vi "connect PG server.vi"(8 "error in (no error)":errorcluster, 11 "SP in":refnum<class "PG messages.lvclass">) -> (0 "error out":errorcluster, 2 "conn_out":u64, 3 "SP out":refnum<class "PG messages.lvclass">)   [LabVIEW 2019, in "PG messages.lvclass"]
uses:
  PG messages.lvclass
  D:/my_projects/projects/Algorithms/Labview/19/Database/Save messages PGserver/Save messages PGserver.lvclass
  Save messages PGserver/Save messages PGserver.lvclass/Save messages PGserver.ctl
  PostgreSQL2LabVIEW/libpqlv/src/PQfinish.vi
  PostgreSQL2LabVIEW/libpqlv/src/PQconnectdb.vi
  PostgreSQL2LabVIEW/libpqlv/src/PQerrorMessage.vi
  PostgreSQL2LabVIEW/libpqlv/src/PQstatus.vi
  <vilib>/dlg_ctls.llb/Space Constant.vi
  PostgreSQL2LabVIEW/libpqUtility/src/PQexecute.vi
  PostgreSQL2LabVIEW/libpqUtility/src/PQlistSequenses.vi
  PostgreSQL2LabVIEW/libpqlv/src/PQresultErrorMessage.vi
  PostgreSQL2LabVIEW/libpqUtility/src/PQclear.vi
  PostgreSQL2LabVIEW/libpqlv/src/PQsendQuery.vi
  PostgreSQL2LabVIEW/libpqlv/src/PQgetResult.vi
  PostgreSQL2LabVIEW/libpqlv/src/PQresultStatus.vi
  PostgreSQL2LabVIEW/libpqUtility/src/PQgetColumn.vi
  PostgreSQL2LabVIEW/libpqlv/src/PQclear.vi
  PostgreSQL2LabVIEW/libpqUtility/src/PQfetchTables.vi
  PostgreSQL2LabVIEW/libpqlv/src/PQgetvalue.vi
  PostgreSQL2LabVIEW/libpqlv/src/PQntuples.vi
  PostgreSQL2LabVIEW/libpqUtility64/libpqutility64.lvlib
  PostgreSQL.lvlib
  Save messages PGserver/Save messages PGserver.lvclass
  PostgreSQL2LabVIEW/libpqUtility/libpqutility.lvlib
panel:
  out "PQStatus":T1(ring)
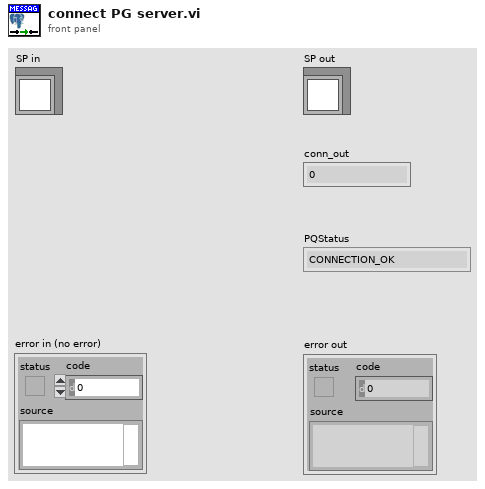
[diagram p1: front panel]
types:
  T1 = enum32{"CONNECTION_OK", "CONNECTION_BAD", "CONNECTION_STARTED", "CONNECTION_MADE", "CONNECTION_AWAITING_RESPONSE", "CONNECTION_AUTH_OK", "CONNECTION_SETENV", "CONNECTION_SSL_STARTUP", "CONNECTION_NEEDED"}
  T2 = typedef "PostgreSQL.lvlib/Coninfo.ctl" = cluster{"host":string, "port":string, "client_encoding":string, "dbname":string, "user":string, "password":string}
  T3 = typedef "Save messages PGserver.lvclass/table parameters.ctl" = cluster{"table postfix":string, "sequence name":string, "columns name":string[], "columns type":string}
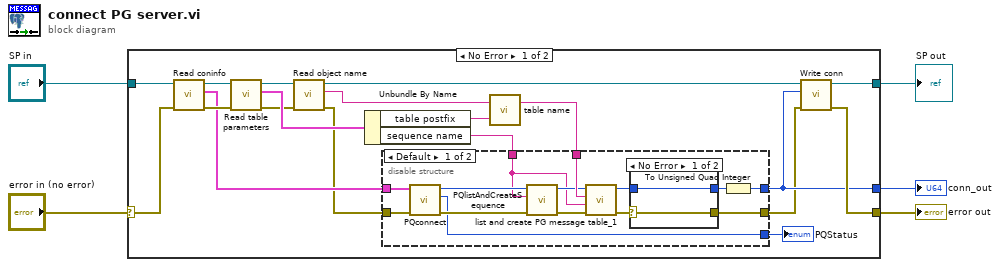
[diagram p0: block diagram]
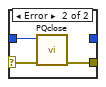
[diagram p2: hidden frame]
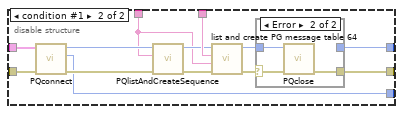
[diagram p3: hidden frame]
diagram:
  n1 = case shown="No Error" "error in (no error)" {
    selector: "error in (no error)" -> [w21 w62]
    tunnel: [w19 w62] -> w4
    tunnel: [w20 w63] -> w2
    tunnel: "SP in" -> [w24 w63]
    tunnel: [w8 _] -> w1
    frame No Error {
      n2 = call "Read coninfo.vi"("error in (no error)"=w21, "SP in"=w24) -> ("error out"=w23:errorcluster, "conninfo"=w10:T2, "SP out"=w22:refnum<class "PG messages.lvclass">)  [unwired: 7 in]
      n3 = call "Read table parameters.vi"("error in (no error)"=w23, "SP in"=w22) -> ("error out"=w12:errorcluster, "table parameters"=w17:T3, "SP out"=w14:refnum<class "PG messages.lvclass">)  [unwired: 7 in]
      n4 = call "Read object name.vi"("error in (no error)"=w12, "SP in"=w14) -> ("error out"=w9:errorcluster, "object name"=w11:string, "SP out"=w13:refnum<class "PG messages.lvclass">)  [unwired: 7 in]
      n5 = Unbundle By Name(w17) -> ("table postfix"=w16:string, "sequence name"=w15:string)
      n6 = call "table name.vi"("postfix"=w16, "object name"=w11) -> ("table name"=w18:string)  [unwired: 1 in]
      n7 = disable-structure shown="Default" {
        disable-tunnel: w18 -> [w38 w56]
        disable-tunnel: w15 -> [w25 w44]
        disable-tunnel: w10 -> [w35 w53]
        disable-tunnel: w9 -> [w34 w52]
        disable-tunnel: [w26 w47] -> w8
        disable-tunnel: [w28 w46] -> w7
        disable-tunnel: [w27 w45] -> w6
        frame condition #0 (active) {
          n8 = call "PQconnect.vi"("error in (no error)"=w34, "conninfo"=w35) -> ("error out"=w32:errorcluster, "PQStatus"=w27:T1, "conn"=w33:u32)  [unwired: 7 in]
          n9 = call "PQlistAndCreateSequence.vi"("error in"=w32, "sequence name"=w25, "conn"=w33) -> ("error out"=w36:errorcluster, "conn_out"=w37:u32)  [unwired: 7 in]
          n10 = call "list and create PG message table_1.vi"("error in"=w36, "serial_n name"=w25, "table name"=w38, "conn"=w37) -> ("error out"=w30:errorcluster, "conn_out"=w31:u32)  [unwired: 6 in]
          n11 = case shown="No Error" w30 {
            selector: w30 -> [w39 w42]
            tunnel: w31 -> [w40 w43]
            tunnel: [w40 _] -> w29
            tunnel: [w39 w41] -> w28
            frame No Error {
            }
            frame Error {
              n12 = call "PQclose.vi"("error in (no error)"=w42, "conn"=w43) -> ("error out"=w41:errorcluster)  [unwired: 9 in]
            }
          }
          n13 = To Unsigned Quad Integer(1:w29) -> (0:w26:u64)
        }
        frame condition #1 {
          n14 = call "PQconnect.vi"("error in (no error)"=w52, "conninfo"=w53) -> ("error out"=w50:errorcluster, "PQStatus"=w45:T1, "conn"=w51:u64)  [unwired: 7 in]
          n15 = call "PQlistAndCreateSequence.vi"("error in"=w50, "sequence name"=w44, "conn"=w51) -> ("error out"=w54:errorcluster, "conn_out"=w55:u64)  [unwired: 7 in]
          n16 = call "list and create PG message table 64.vi"("error in"=w54, "serial_n name"=w44, "table name"=w56, "conn"=w55) -> ("error out"=w48:errorcluster, "conn_out"=w49:u64)  [unwired: 6 in]
          n17 = case shown="Error" w48 {
            selector: w48 -> [w57 w60]
            tunnel: w49 -> [w58 w61]
            tunnel: [w58 _] -> w47
            tunnel: [w57 w59] -> w46
            frame No Error {
            }
            frame Error {
              n18 = call "PQclose.vi"("error in (no error)"=w60, "conn"=w61) -> ("error out"=w59:errorcluster)  [unwired: 9 in]
            }
          }
        }
      }
      "PQStatus" <- w6
      n19 = call "Write conn.vi"("error in (no error)"=w7, "conn"=w8, "SP in"=w13) -> ("error out"=w19:errorcluster, "SP out"=w20:refnum<class "PG messages.lvclass">)  [unwired: 7 in]
    }
    frame Error {
    }
  }
  "error out" <- w4
  "SP out" <- w2
  "conn_out" <- w1
